vi "ButtonEnableAutoStack.vi"(10 "POVs":i16[](array[numeric]), 11 "Buttons":bool[](array[boolean])) -> ()   [LabVIEW 2014]
uses:
  AutomationGlobals.vi
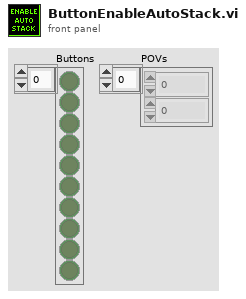
[diagram p1: front panel]
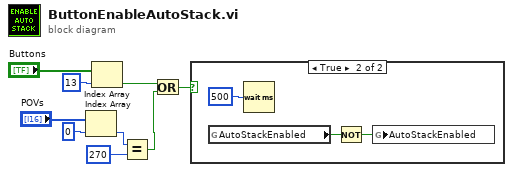
[diagram p0: block diagram]
diagram:
  n1 = Index Array(array="POVs", index=0) -> (element=w3:i16)
  n2 = Index Array(array="Buttons", index=13) -> (element=w7:bool)
  n3 = Equal?(x=w3, y=i16 270) -> (x = y?=w2:bool)
  n4 = Or(x=w7, y=w2) -> (x .or. y?=w4:bool)
  n5 = case shown="True" w4 {
    frame False {
    }
    frame True {
      n6 = global read "AutomationGlobals.vi" "AutoStackEnabled"() -> (w12:bool)
      n7 = Wait (ms)(milliseconds to wait=u32 500) -> ()  [unwired: 1 out]
      n8 = Not(x=w12) -> (.not. x?=w11:bool)
      n9 = global write "AutomationGlobals.vi" "AutoStackEnabled"(w11) -> ()
    }
  }
